vi "SVPO Envelope Detection (1 Ch DBL WDT) with IC.vi"(0 "scaled signal [EU]":waveform(dbl)={"t0"=timestamp(0 s since 1904-01-01), "dt"=0.0, "Y"=[]}, 1 "reset? (F)":bool, 9 "band specification":T3={"center frequency [Hz]"=4800.0, "span [Hz]"=2000.0}, 11 "initial conditions":T1 {"filter settings"."filters"."coefficients" format="%.2f"}) -> (4 "envelope signal [EU]":waveform(dbl), 15 "final conditions":T1 {"filter settings"."filters"."coefficients" format="%.2f"})   [LabVIEW 2017, in "SoundVib_FaultAnalysis.lvlib"]
doc: "Extracts the modulating signal, or envelope signal, from an amplitude-modulated signal. You can use the envelope detection technique to identify the mechanical faults that have amplitude-modulating effect on the vibration signal of a machine. Use this VI on embedded targets that have limited computational resources. Wire data to the <B>scaled signal [EU]</B> input to determine the polymorphic instance to use or manually select the instance."
uses:
  <vilib>/addons/Sound and Vibration/Order Analysis/Fault Analysis/SoundVib_FaultAnalysis.lvlib
  <vilib>/addons/_NISVFA/_Shared subVIs/Controls/svc_Envelope Detection State.ctl
  <vilib>/addons/_NISVFA/_Shared subVIs/Controls/OAT Decimation Filter.ctl
  <vilib>/addons/Sound and Vibration/Order Analysis/Resample Order Tracking/SubVIs/oa_Calculate CIC Decimation Filter Coefficients.vi
  <vilib>/addons/Sound and Vibration/Order Analysis/Fault Analysis/SubVIs/sv_Compute Shift and Low Pass Filter with IC.vi
  <vilib>/addons/Sound and Vibration/Order Analysis/Resample Order Tracking/SubVIs/OAT Frequency Shift (Mixer).vi
  <vilib>/addons/Sound and Vibration/Order Analysis/Resample Order Tracking/SubVIs/oa_Decimation with CIC and Compensation Filter.vi
  <vilib>/addons/Sound and Vibration/Order Analysis/Fault Analysis/SubVIs/oa_Demodulation Initial States (1 Channel).vi
  <vilib>/addons/Sound and Vibration/Order Analysis/Adv Resampling/OAT Single Stage Decimation with IC.vi
  <vilib>/addons/Sound and Vibration/Order Analysis/Resample Order Tracking/SubVIs/OAT CIC Decimation.vi
  <vilib>/addons/Sound and Vibration/Order Analysis/Resample Order Tracking/SubVIs/oa_Interpolate Zeros Between Samples.vi
  <vilib>/addons/Sound and Vibration/Order Analysis/Resample Order Tracking/SubVIs/oa_Calculate Delay of CIC Decimation Interpolation Filter.vi
  <vilib>/addons/Sound and Vibration/Order Analysis/Resample Order Tracking/SubVIs/oa_Create CIC Compensation Filter.vi
  <vilib>/addons/Sound and Vibration/Order Analysis/Resample Order Tracking/SubVIs/oa_Create CIC LP Truncation Filter.vi
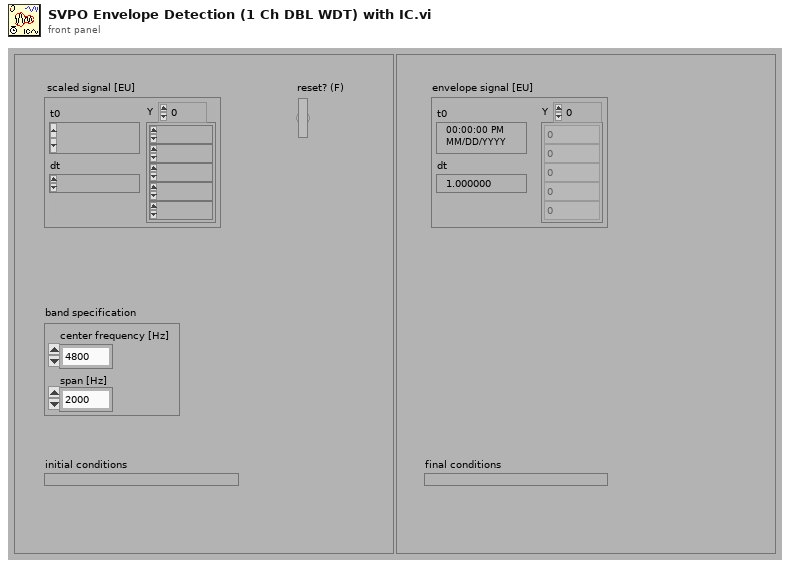
[diagram p1: front panel]
types:
  T1 = typedef "svc_Envelope Detection State.ctl" = cluster{"filter settings":cluster{"CIC Settings":cluster{"Numeric":i32, i32, i32}, "filters":T2[], "delay":i32, "interpolation factor":i32}, "filter state":cluster{"t0":dbl, "phase":dbl, "real filter state":cluster{cluster{dbl[]}, cluster{dbl[]}[]}, "imaginary filter state":cluster{cluster{dbl[]}, cluster{dbl[]}[]}, "delay":i32}, "reset pending":bool}
  T2 = typedef "OAT Decimation Filter.ctl" = cluster{"coefficients":dbl[], "factor":i32}
  T3 = cluster{"center frequency [Hz]":dbl, "span [Hz]":dbl}
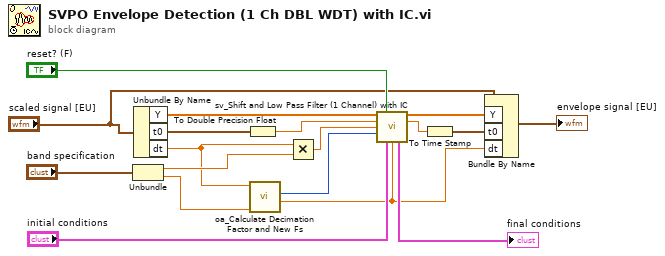
[diagram p0: block diagram]
diagram:
  n1 = Unbundle("band specification") -> ("center frequency [Hz]"=w7:dbl, "span [Hz]"=w8:dbl)
  n2 = Unbundle By Name("scaled signal [EU]") -> ("Y"=w13:dbl[], "t0"=w9:timestamp, "dt"=w6:dbl)
  n3 = To Double Precision Float(number=w9) -> (double precision float=w12:dbl)
  n4 = call <vilib>:"oa_Calculate Decimation Factor and New Fs.vi"("span"=w8, "dt"=w6) -> ("new dt"=w1:dbl, "decimation factor"=w15:i32)  [unwired: 8 in]
  n5 = Multiply(x=w6, y=w7) -> (x*y=w16:dbl)
  n6 = call <vilib>:"sv_Shift and Low Pass Filter (1 Channel) with IC.vi"("input signal"=w13, "reset? (F)"="reset? (F)", "t0"=w12, "center"=w16, "decimation factor"=w15, "initial conditions"="initial conditions", "new dt"=w1) -> ("enveloped signal"=w14:dbl[], "t0 out"=w11:dbl, "final conditions"=→"final conditions":T1)  [unwired: 5 in, 1 out]
  n7 = To Time Stamp(1:w11) -> (0:w10:timestamp)
  n8 = Bundle By Name(cluster="scaled signal [EU]", "Y"=w14, "t0"=w10, "dt"=w1) -> (→"envelope signal [EU]":waveform(dbl))
